vi "RotationBlocking_(SubVI).vi"(3 "Min/Max Yaw Steps":i32, 4 "Yaw Step Amount":i32, 5 "Min/Max Pitch Steps":i32, 6 "Pitch Step Amount":i32) -> (0 "Yaw Array":i32[](array[numeric]), 1 "Pitch Array":i32[](array[numeric]), 2 "Numeric":dbl=1.8)   [LabVIEW 2010]
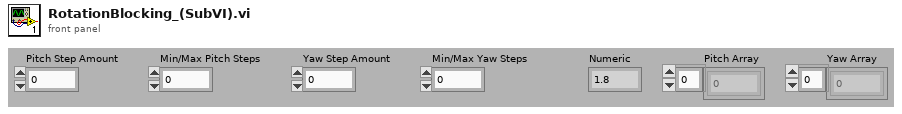
[diagram p1: front panel]
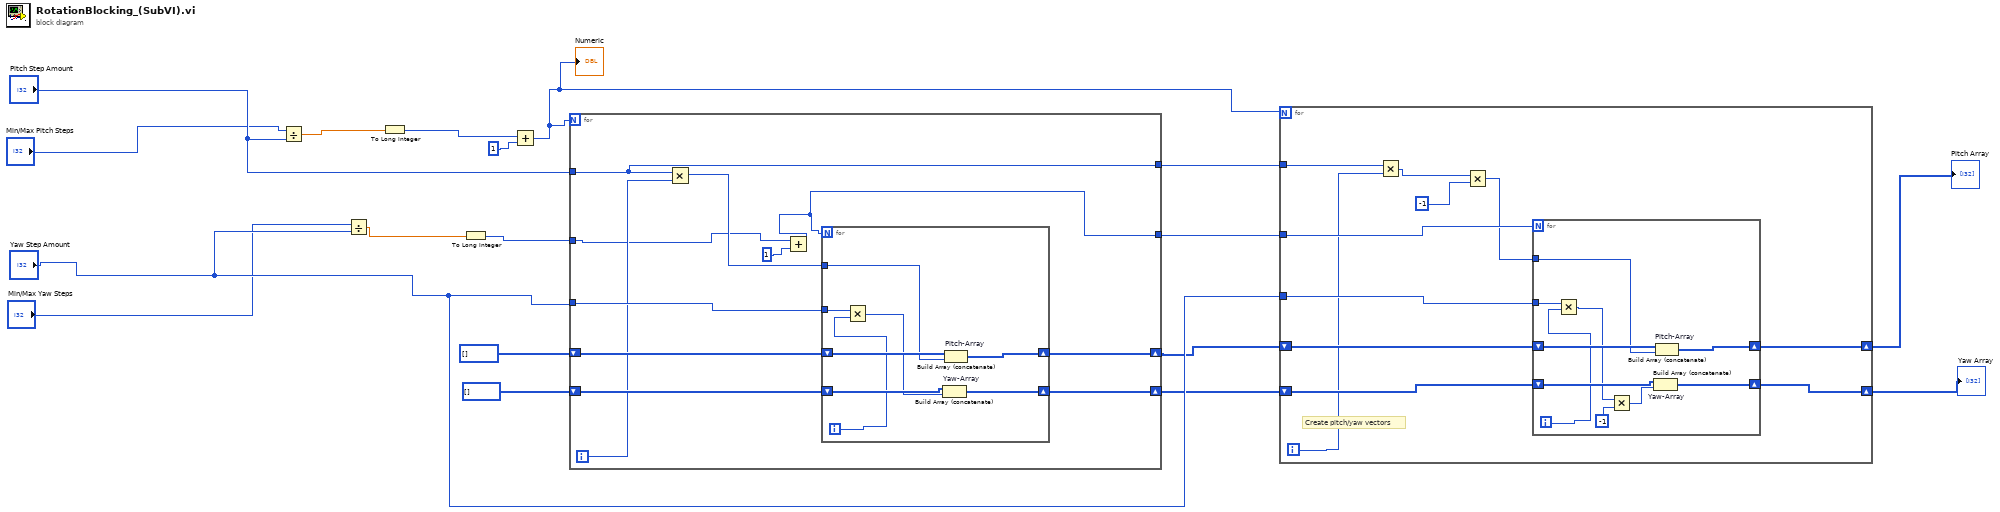
[diagram p0: block diagram]
diagram:
  # "Create pitch/yaw vectors"
  n1 = Divide(x="Min/Max Pitch Steps", y="Pitch Step Amount") -> (x/y=w15:dbl)
  n2 = Divide(x="Min/Max Yaw Steps", y="Yaw Step Amount") -> (x/y=w18:dbl)
  n3 = To Long Integer(number=w15) -> (32bit integer=w16:i32)
  n4 = To Long Integer(number=w18) -> (32bit integer=w17:i32)
  n5 = Add(x=w16, y=1) -> (x+y=w14:i32)
  "Numeric" <- w14
  n6 = for {
    N: w14 -> [_]
    shift-right: [w28] -> w6
    shift-left: i32[] [] -> [w29]
    shift-right: [w26] -> w5
    shift-left: i32[] [] -> [w27]
    tunnel: "Pitch Step Amount" -> [w23]
    tunnel: "Yaw Step Amount" -> [w25]
    tunnel: [w19] -> w4
    tunnel: [w23] -> w3
    tunnel: w17 -> [w20]
    i -> [w21]
    n7 = Multiply(x=w23, y=w21) -> (x*y=w24:i32)
    n8 = Add(x=w20, y=1) -> (x+y=w19:i32)
    n9 = for {
      N: w19 -> [_]
      shift-right: [w37] -> w28
      shift-left: w29 -> [w36]
      shift-right: [w34] -> w26
      shift-left: w27 -> [w35]
      tunnel: w25 -> [w33]
      tunnel: w24 -> [w31]
      i -> [w30]
      n10 = Multiply(x=w33, y=w30) -> (x*y=w32:i32)
      n11 = Build Array (concatenate) "Yaw-Array"(w35, w32) -> (w34:i32[])
      n12 = Build Array (concatenate) "Pitch-Array"(w36, w31) -> (w37:i32[])
    }
  }
  n13 = for {
    N: w14 -> [_]
    shift-right: [w47] -> w1
    shift-left: w6 -> [w48]
    shift-right: [w45] -> w2
    shift-left: w5 -> [w46]
    tunnel: w4 -> [w44]
    tunnel: w3 -> [w43]
    tunnel: "Yaw Step Amount" -> [w42]
    i -> [w38]
    n14 = Multiply(x=w43, y=w38) -> (x*y=w41:i32)
    n15 = Multiply(x=w41, y=-1) -> (x*y=w40:i32)
    n16 = for {
      N: w44 -> [_]
      shift-right: [w58] -> w47
      shift-left: w48 -> [w57]
      shift-right: [w55] -> w45
      shift-left: w46 -> [w56]
      tunnel: w42 -> [w54]
      tunnel: w40 -> [w53]
      i -> [w49]
      n17 = Multiply(x=w54, y=w49) -> (x*y=w51:i32)
      n18 = Multiply(x=w51, y=-1) -> (x*y=w52:i32)
      n19 = Build Array (concatenate) "Yaw-Array"(w56, w52) -> (w55:i32[])
      n20 = Build Array (concatenate) "Pitch-Array"(w57, w53) -> (w58:i32[])
    }
  }
  "Yaw Array" <- w2
  "Pitch Array" <- w1
